vi "TERMINAL.vi"(0 "Indicateur Refnum":refnum<vi>, 1 "Terminal Refnum":refnum<vi>, 2 "Indicateur d'état":string="WTF ?!?") -> ()   [LabVIEW 2011]
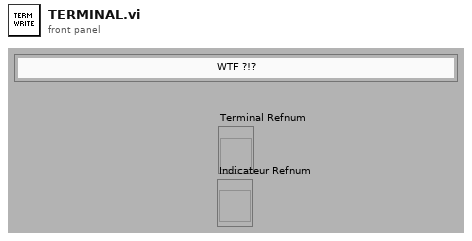
[diagram p1: front panel]
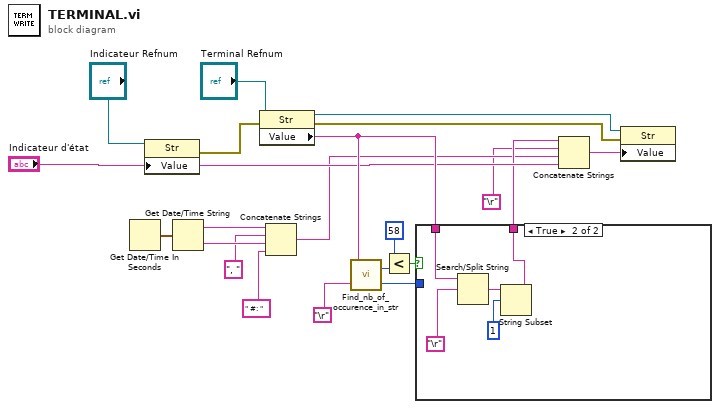
[diagram p0: block diagram]
diagram:
  n1 = Get Date/Time In Seconds() -> (seconds since 1Jan1904=w15:timestamp)
  n2 = property class="Str"(reference="Indicateur Refnum", "Value"="Indicateur d'état") -> (error out=w17:errorcluster)  [unwired: 1 in, 1 out]
  n3 = Get Date/Time String(seconds (now)=w15) -> (date string=w9:string, time string=w8:string)  [unwired: 2 in]
  n4 = property class="Str"(reference="Terminal Refnum", error in=w17) -> (reference out=w19:refnum<vi>, error out=w18:errorcluster, "Value"=w12:string)
  n5 = Concatenate Strings(w9, ", ", w8, " #: ") -> (w2:string)
  n6 = call "Find_nb_of_occurence_in_str.vi"("search string/char"="\r", "Str In"=w12) -> ("Index"=w13:i32, "Nb of occurrence"=w11:i32)
  n7 = Less?(x=58, y=w11) -> (x < y?=w10:bool)
  n8 = case shown="True" w10 {
    tunnel: w13 -> [_ _]
    tunnel: w12 -> [w22 w27]
    tunnel: [w22 w23] -> w3
    frame False {
    }
    frame True {
      n9 = Search/Split String(string=w27, search string/char (-)="\r") -> (match + rest of string=w25:string)  [unwired: 1 in, 2 out]
      n10 = String Subset(string=w25, offset (0)=1) -> (substring=w23:string)  [unwired: 1 in]
    }
  }
  n11 = Concatenate Strings(w3, "\r", w2, "Indicateur d'état") -> (w21:string)
  n12 = property class="Str"(reference=w19, error in=w18, "Value"=w21) -> ()  [unwired: 2 out]
